vi "Get_right_exp.vi"(8 "error in (no error)":errorcluster, 11 "Control-Client in":refnum<class "Control-Client.lvclass">) -> (0 "error out":errorcluster, 2 "Right experiment":refnum<class "Experiment.lvclass">, 3 "Control-Client out":refnum<class "Control-Client.lvclass">)   [LabVIEW 2019, in "Control-Client.lvclass"]
uses:
  Control-Client.lvclass
  Experiments/Experiment.lvclass
  Control-Client.lvclass/Control-Client.ctl
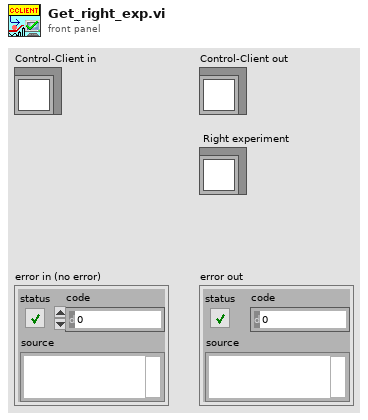
[diagram p1: front panel]
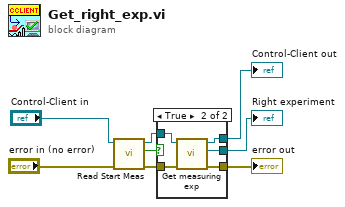
[diagram p0: block diagram]
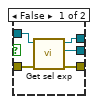
[diagram p2: hidden frame]
diagram:
  n1 = call "Read Start Meas.vi"("error in (no error)"="error in (no error)", "Control-Client in"="Control-Client in") -> ("error out"=w7:errorcluster, "Start Meas"=w8:bool, "Control-Client out"=w6:refnum<class "Control-Client.lvclass">)  [unwired: 7 in]
  n2 = case shown="True" w8 {
    tunnel: [w13 w17] -> w1
    tunnel: [w12 w18] -> w2
    tunnel: [w11 w16] -> w3
    tunnel: w6 -> [w10 w14]
    tunnel: w7 -> [w9 w15]
    frame False {
      n3 = call "Get sel exp.vi"("error in (no error)"=w9, "Control-Client in"=w10) -> ("error out"=w11:errorcluster, "Sel experiment"=w12:refnum<class "Experiment.lvclass">, "Control-Client out"=w13:refnum<class "Control-Client.lvclass">)  [unwired: 7 in]
    }
    frame True {
      n4 = call "Get measuring exp.vi"("error in (no error)"=w15, "Control-Client in"=w14) -> ("error out"=w16:errorcluster, "Measured experiment"=w18:refnum<class "Experiment.lvclass">, "Control-Client out"=w17:refnum<class "Control-Client.lvclass">)  [unwired: 7 in]
    }
  }
  "error out" <- w3
  "Right experiment" <- w2
  "Control-Client out" <- w1
